vi "_Chain Mapping Map.vi"(11 "Messages of Chain Nodes":T1(array[cluster])) -> (1 "Variant":variant=variant("action1"=variant(string "X$3"), "action2"=variant(string "X$1"), "action3"=variant(string "X$2"), "action4"=variant(string "X$1")), 3 "Messages of Chain Nodes (Dup)":T1(array[cluster]))   [LabVIEW 2017, in "Communicable State Machine.lvlib"]
uses:
  Communicable State Machine.lvlib
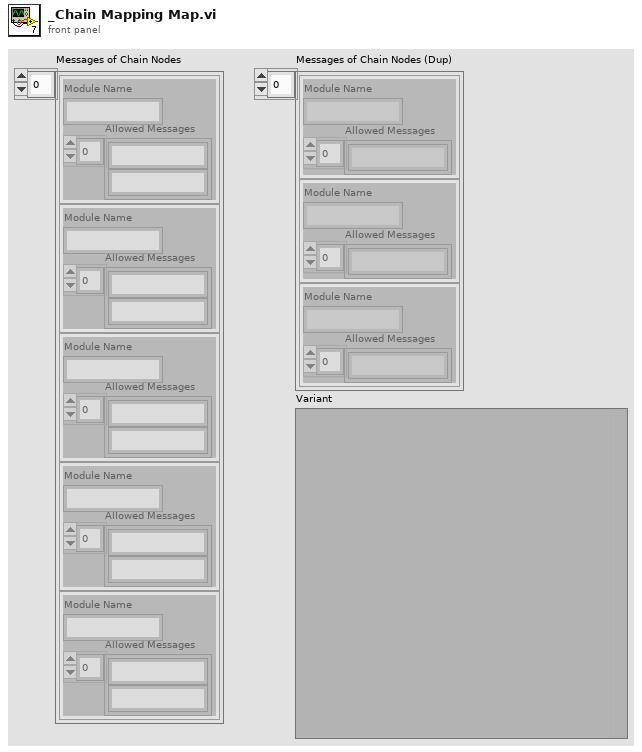
[diagram p1: front panel]
types:
  T1 = cluster{"Module Name":string, "Allowed Messages":string[]}[]
  T2 = cluster{"Module Name":string, "Allowed Messages":string[]}
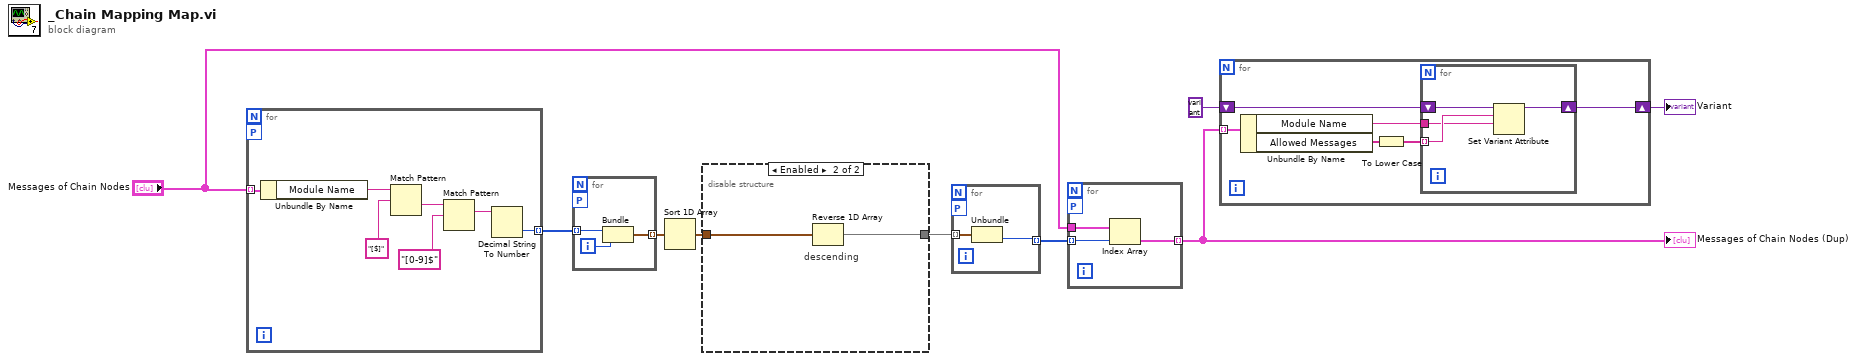
[diagram p0: block diagram]
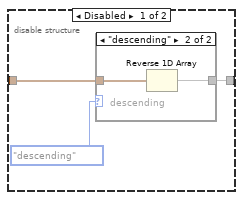
[diagram p2: hidden frame]
diagram:
  n1 = for {
    tunnel: "Messages of Chain Nodes" -> [w16] mode=indexing
    tunnel: [w10] -> w9 mode=indexing
    workers-P: _ -> [_]
    n2 = Unbundle By Name(w16) -> ("Module Name"=w15:string)
    n3 = Match Pattern(string=w15, regular expression="[$]") -> (after substring=w13:string)  [unwired: 1 in, 3 out]
    n4 = Match Pattern(string=w13, regular expression="[0-9]$") -> (match substring=w11:string)  [unwired: 1 in, 3 out]
    n5 = Decimal String To Number(string=w11) -> (number=w10:i32)  [unwired: 2 in, 1 out]
  }
  n6 = for {
    tunnel: w9 -> [w19] mode=indexing
    tunnel: [w17] -> w5 mode=indexing
    workers-P: _ -> [_]
    i -> [w18]
    n7 = Bundle(w19, w18) -> (w17:cluster{i32, i32})  [unwired: 1 in]
  }
  n8 = Sort 1D Array(array=w5) -> (sorted array=w6:cluster{i32, i32}[])
  n9 = disable-structure shown="Enabled" {
    disable-tunnel: w6 -> [w21 w27]
    disable-tunnel: [w20 w26] -> w4
    frame Disabled {
      n10 = case shown="\"descending\"" enum16{"ascending", "descending"}."descending" ("Order") {
        tunnel: [w23 w24] -> w20
        tunnel: w21 -> [w23 w25]
        frame "ascending", Default {
        }
        frame "descending" {
          # "descending"
          n11 = Reverse 1D Array(array=w25) -> (reversed array=w24:cluster{i32, i32}[])
        }
      }
    }
    frame Enabled {
      # "descending"
      n12 = Reverse 1D Array(array=w27) -> (reversed array=w26:cluster{i32, i32}[])
    }
  }
  n13 = for {
    tunnel: w4 -> [w29] mode=indexing
    tunnel: [w28] -> w8 mode=indexing
    workers-P: _ -> [_]
    n14 = Unbundle(w29) -> (w28:i32)  [unwired: 1 out]
  }
  n15 = for {
    tunnel: w8 -> [w32] mode=indexing
    tunnel: "Messages of Chain Nodes" -> [w31]
    tunnel: [w30] -> w3 mode=indexing
    workers-P: _ -> [_]
    n16 = Index Array(array=w31, index=w32) -> (element=w30:T2)
  }
  "Messages of Chain Nodes (Dup)" <- w3
  n17 = for {
    tunnel: w3 -> [w36] mode=indexing
    shift-right: [w37] -> w1
    shift-left: variant ("variant") -> [w38]
    n18 = Unbundle By Name(w36) -> ("Module Name"=w34:string, "Allowed Messages"=w35:string[])
    n19 = To Lower Case(string=w35) -> (all lower case string=w33:string[])
    n20 = for {
      shift-right: [w41] -> w37
      shift-left: w38 -> [w42]
      tunnel: w33 -> [w40] mode=indexing
      tunnel: w34 -> [w39]
      n21 = Set Variant Attribute(Variant=w42, name=w40, value=w39) -> (Variant out=w41:variant)  [unwired: 1 in, 2 out]
    }
  }
  "Variant" <- w1
